vi "Wyswietlanie_danych (SubVI).vi"(7 "unsigned byte array":u8[](array[numeric])) -> (8 "X":dbl(slide) scale=0.0..360.0, 9 "Akc X":dbl format="%.2f", 10 "¯yro X":u32, 12 "Y":dbl(slide) scale=0.0..360.0, 13 "Akc Y":dbl format="%.2f", 14 "¯yro Y":u32, 16 "Z":dbl(slide) scale=0.0..360.0, 17 "Akc Z":dbl format="%.2f", 18 "¯yro Z":u32)   [LabVIEW 2012]
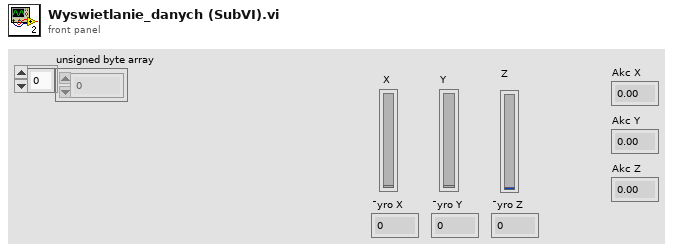
[diagram p1: front panel]
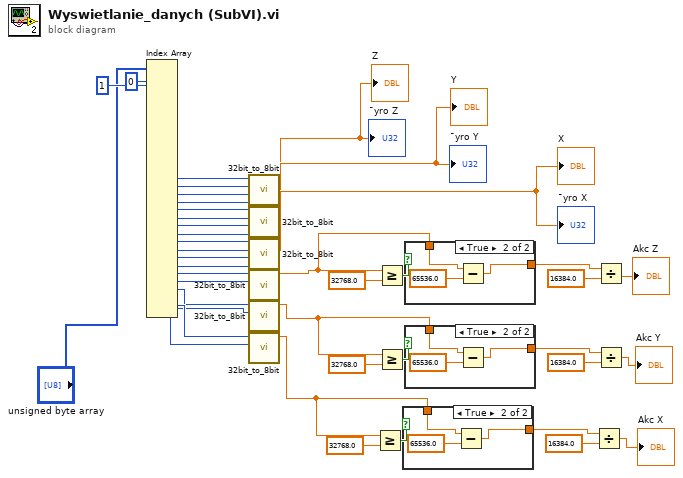
[diagram p0: block diagram]
diagram:
  n1 = Index Array(array="unsigned byte array", index #1=0 ("index"), index #2=1 ("index")) -> (element #13=w22:u8, element #14=w23:u8, element #15=w24:u8, element #16=w25:u8, element #17=w26:u8, element #18=w27:u8, element #19=w28:u8, element #20=w29:u8, element #21=w30:u8, element #22=w31:u8, element #23=w32:u8, element #24=w33:u8, element #25=w37:u8, element #26=w38:u8, element #27=w39:u8, element #28=w40:u8, element #29=w41:u8, element #30=w42:u8)  [unwired: 28 in, 12 out]
  n2 = call "32bit_to_8bit.vi"("Numeric 6"=w25, "Numeric 5"=w24, "Numeric 4"=w23, "Numeric in"=w22) -> ("Numeric out"=→"¯yro Z" →"Z":dbl)  [unwired: 6 in, 1 out]
  n3 = call "32bit_to_8bit.vi"("Numeric 6"=w29, "Numeric 5"=w28, "Numeric 4"=w27, "Numeric in"=w26) -> ("Numeric out"=→"¯yro Y" →"Y":dbl)  [unwired: 6 in, 1 out]
  n4 = call "32bit_to_8bit.vi"("Numeric 6"=w33, "Numeric 5"=w32, "Numeric 4"=w31, "Numeric in"=w30) -> ("Numeric out"=→"¯yro X" →"X":dbl)  [unwired: 6 in, 1 out]
  n5 = call "32bit_to_8bit.vi"("Numeric 4"=w38, "Numeric in"=w37) -> ("Numeric 3"=w15:dbl)  [unwired: 8 in, 1 out]
  n6 = call "32bit_to_8bit.vi"("Numeric 4"=w40, "Numeric in"=w39) -> ("Numeric 3"=w9:dbl)  [unwired: 8 in, 1 out]
  n7 = call "32bit_to_8bit.vi"("Numeric 4"=w42, "Numeric in"=w41) -> ("Numeric 3"=w4:dbl)  [unwired: 8 in, 1 out]
  n8 = Greater Or Equal?(x=w4, y=32768.0) -> (x >= y?=w6:bool)
  n9 = Greater Or Equal?(x=w15, y=32768.0) -> (x >= y?=w16:bool)
  n10 = Greater Or Equal?(x=w9, y=32768.0) -> (x >= y?=w11:bool)
  n11 = case shown="True" w6 {
    tunnel: w4 -> [w43 w45]
    tunnel: [w43 w44] -> w5
    frame False {
    }
    frame True {
      n12 = Subtract(x=w45, y=65536.0) -> (x-y=w44:dbl)
    }
  }
  n13 = case shown="True" w16 {
    tunnel: w15 -> [w47 w49]
    tunnel: [w47 w48] -> w14
    frame False {
    }
    frame True {
      n14 = Subtract(x=w49, y=65536.0) -> (x-y=w48:dbl)
    }
  }
  n15 = case shown="True" w11 {
    tunnel: w9 -> [w51 w53]
    tunnel: [w51 w52] -> w10
    frame False {
    }
    frame True {
      n16 = Subtract(x=w53, y=65536.0) -> (x-y=w52:dbl)
    }
  }
  n17 = Divide(x=w5, y=16384.0) -> (x/y=→"Akc X":dbl)
  n18 = Divide(x=w14, y=16384.0) -> (x/y=→"Akc Z":dbl)
  n19 = Divide(x=w10, y=16384.0) -> (x/y=→"Akc Y":dbl)
